vi "CRYGet Harmonics Curve array.vi"(4 "Impedance and Mic Current In":bool[](array[boolean]), 5 "Additive Info":T4, 6 "Option Array In":bool[](array[boolean]), 7 "Unit Info":T5, 8 "Diff array":dbl[](array[numeric]), 9 "IM array":dbl[](array[numeric]), 10 "Harmonics array":dbl[](array[numeric]), 11 "Type":u16) -> (0 "Display Array":T3(array[cluster]), 1 "Unit Info Out":T2[](array[typedef]), 2 "Harmonics Orders Out":dbl[](array[numeric]), 3 "Curve Info Array Out":T1)   [LabVIEW 2013]
uses:
  Typedef Control/CRYUnit Info Cluster.ctl
  Typedef Control/CRYUnit Info Out Cluster.ctl
  Typedef Control/CRYAnalysis CurveName Cluster.ctl
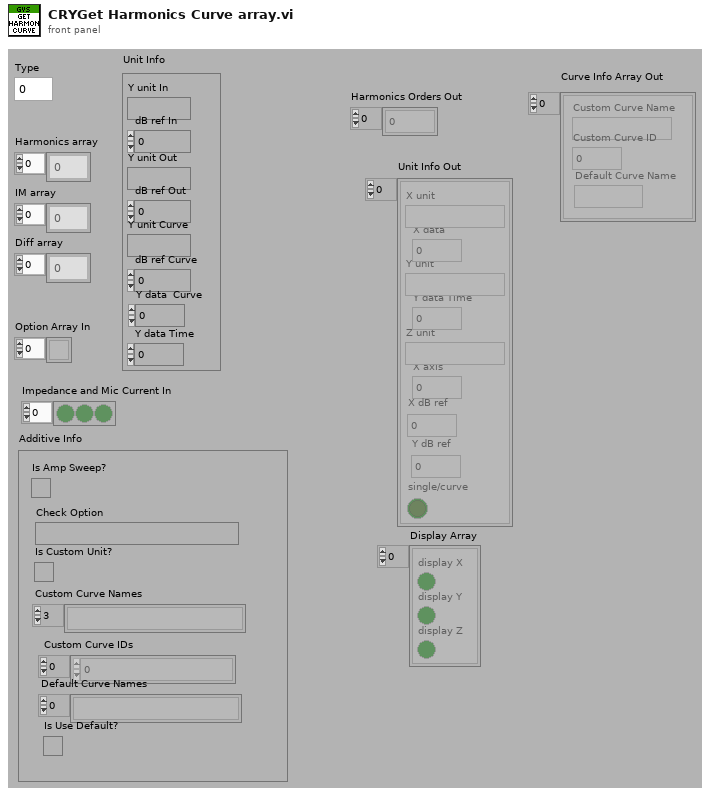
[diagram p1: front panel]
types:
  T1 = typedef "CRYAnalysis CurveName Cluster.ctl" = cluster{"Custom Curve Name":string, "Custom Curve ID":i32, "Default Curve Name":string}[]
  T2 = typedef "CRYUnit Info Out Cluster.ctl" = cluster{"X unit":string, "X data":u16, "Y unit":string, "Y data Time":u16, "Z unit":string, "X axis":u16, "X dB ref":dbl, "Y dB ref":dbl, "single/curve":bool}
  T3 = cluster{"display X":bool, "display Y":bool, "display Z":bool}[]
  T4 = cluster{"Is Amp Sweep?":bool, "Check Option":string, "Is Custom Unit?":bool, "Custom Curve Names":string[], "Custom Curve IDs":i32[], "Default Curve Names":string[], "Is Use Default?":bool}
  T5 = typedef "CRYUnit Info Cluster.ctl" = cluster{"Y unit In":string, "dB ref In":dbl, "Y unit Out":string, "dB ref Out":dbl, "Y unit Curve":string, "dB ref Curve":dbl, "Y data  Curve":u16, "Y data Time":u16}
  T6 = enum32{"English", "Chinese", "Korean", "Japanese", "Russian", "Chinese traditional"}
  T7 = cluster{"Y unit Out":string, "dB":u16, "Y unit Curve":string, "Y data  Curve":u16, "Y unit Curve":string, "Lin":u16, "dB ref Out":dbl, "dB ref Curve":dbl, "display X":bool}
  T8 = cluster{"display X":bool, "display Y":bool, "display Z":bool}
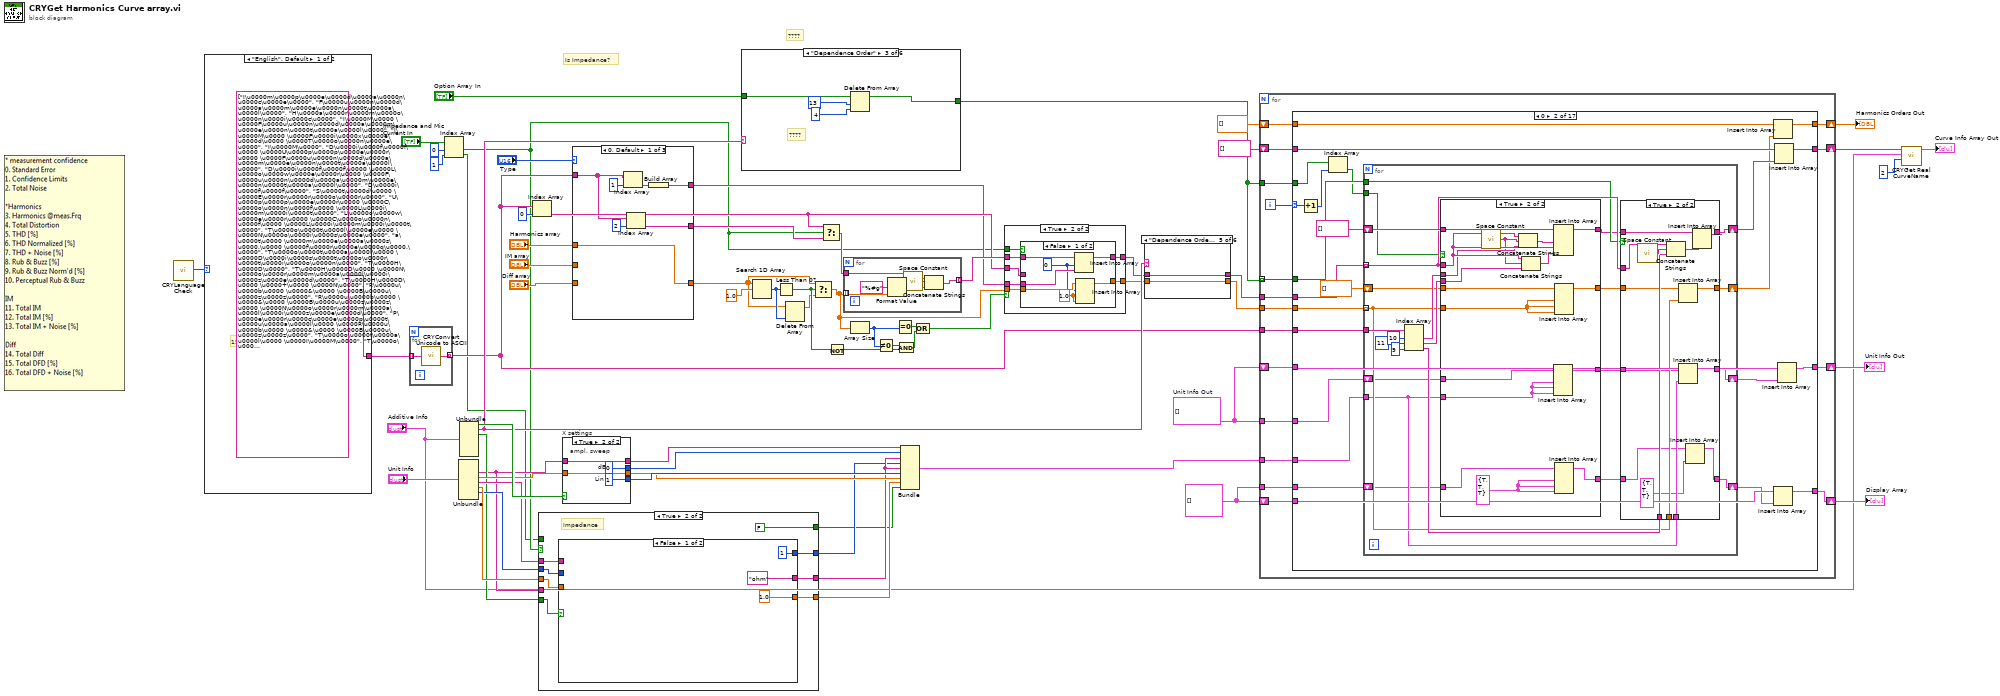
[diagram p0: block diagram]
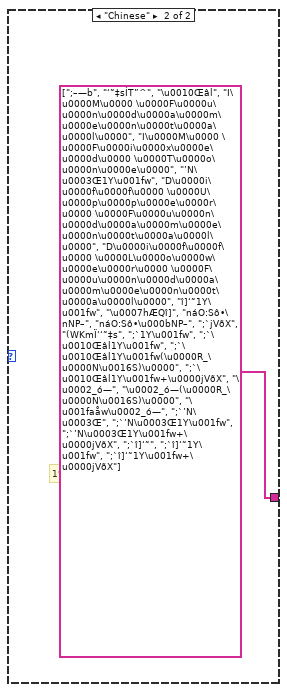
[diagram p2: hidden frame]
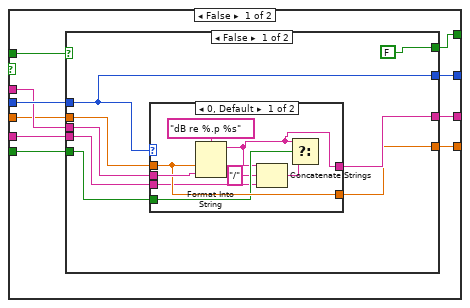
[diagram p3: hidden frame]
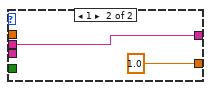
[diagram p4: hidden frame]
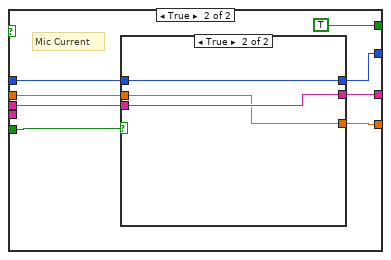
[diagram p5: hidden frame]
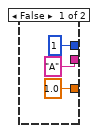
[diagram p6: hidden frame]
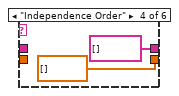
[diagram p11: hidden frame]
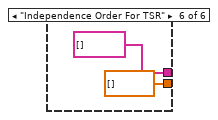
[diagram p12: hidden frame]
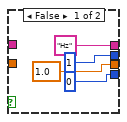
[diagram p13: hidden frame]
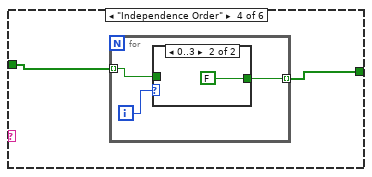
[diagram p16: hidden frame]
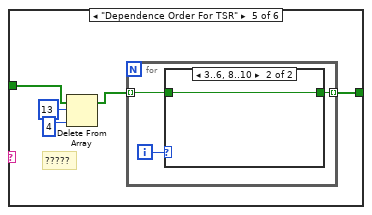
[diagram p18: hidden frame]
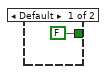
[diagram p19: hidden frame]
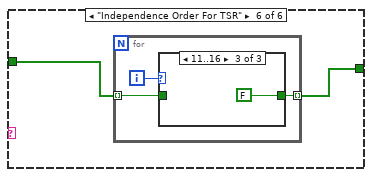
[diagram p20: hidden frame]
diagram:
  w28 = T3 [] ("Display Array")
  w31 = T2[] []  # Unit Info Out
  # "????"
  # "Is Impedance?"
  n1 = call "CRYLanguage Check.vi"() -> ("Language"=w8:T6)  [unwired: 10 in, 1 out]
  n2 = case shown="\"English\", Default" w8 {
    tunnel: [string[] ["I\u0000m\u0000p\u0000e\u0000d\u0000a\u0000n\u0000c\u0000e\u0000", "F\u0000u\u0000n\u0000d\u0000a\u0000m\u0000e\u0000n\u0000t\u0000a\u0000l\u0000", "H\u0000a\u0000r\u0000m\u0000o\u0000n\u0000i\u0000c\u0000", "I\u0000M\u0000 \u0000F\u0000u\u0000n\u0000d\u0000a\u0000m\u0000e\u0000n\u0000t\u0000a\u0000l\u0000", "I\u0000M\u0000 \u0000F\u0000i\u0000x\u0000e\u0000d\u0000 \u0000T\u0000o\u0000n\u0000e\u0000", "I\u0000M\u0000", "D\u0000i\u0000f\u0000f\u0000 \u0000U\u0000p\u0000p\u0000e\u0000r\u0000 \u0000F\u0000u\u0000n\u0000d\u0000a\u0000m\u0000e\u0000n\u0000t\u0000a\u0000l\u0000", "D\u0000i\u0000f\u0000f\u0000 \u0000L\u0000o\u0000w\u0000e\u0000r\u0000 \u0000F\u0000u\u0000n\u0000d\u0000a\u0000m\u0000e\u0000n\u0000t\u0000a\u0000l\u0000", "D\u0000i\u0000f\u0000f\u0000", "S\u0000t\u0000d\u0000 \u0000E\u0000r\u0000r\u0000o\u0000r\u0000", "U\u0000p\u0000p\u0000e\u0000r\u0000 \u0000C\u0000o\u0000n\u0000f\u0000 \u0000L\u0000i\u0000m\u0000i\u0000t\u0000", "L\u0000o\u0000w\u0000e\u0000r\u0000 \u0000C\u0000o\u0000n\u0000f\u0000 \u0000L\u0000i\u0000m\u0000i\u0000t\u0000", "T\u0000o\u0000t\u0000l\u0000e\u0000 \u0000N\u0000o\u0000i\u0000s\u0000e\u0000", "a\u0000t\u0000 \u0000m\u0000e\u0000a\u0000s\u0000.\u0000 \u0000f\u0000r\u0000e\u0000q\u0000.\u0000", "T\u0000o\u0000t\u0000a\u0000l\u0000 \u0000D\u0000i\u0000s\u0000t\u0000o\u0000r\u0000t\u0000i\u0000o\u0000n\u0000", "T\u0000H\u0000D\u0000", "T\u0000H\u0000D\u0000 \u0000N\u0000o\u0000r\u0000m\u0000a\u0000l\u0000i\u0000z\u0000e\u0000d\u0000", "T\u0000H\u0000D\u0000 \u0000+\u0000 \u0000N\u0000", "R\u0000u\u0000b\u0000 \u0000&\u0000 \u0000B\u0000u\u0000z\u0000z\u0000", "R\u0000u\u0000b\u0000 \u0000&\u0000 \u0000B\u0000u\u0000z\u0000z\u0000 \u0000N\u0000o\u0000r\u0000m\u0000a\u0000l\u0000i\u0000z\u0000e\u0000d\u0000", "P\u0000e\u0000r\u0000c\u0000e\u0000p\u0000t\u0000u\u0000a\u0000l\u0000 \u0000R\u0000u\u0000b\u0000 \u0000&\u0000 \u0000B\u0000u\u0000z\u0000z\u0000", "T\u0000o\u0000t\u0000a\u0000l\u0000 \u0000I\u0000M\u0000", "T\u0000o\u0000t\u0000a\u0000l\u0000 \u0000I\u0000M\u0000D\u0000", "T\u0000o\u0000t\u0000a\u0000l\u0000 \u0000I\u0000M\u0000D\u0000 \u0000+\u0000 \u0000N\u0000", "T\u0000o\u0000t\u0000a\u0000l\u0000 \u0000D\u0000i\u0000f\u0000f\u0000", "T\u0000o\u0000t\u0000a\u0000l\u0000 \u0000D\u0000F\u0000D\u0000", "T\u0000o\u0000t\u0000a\u0000l\u0000 \u0000D\u0000F\u0000D\u0000 \u0000+\u0000 \u0000N\u0000"] ("Array") string[] [";–—b", "‘˜‡sÍT”^", "\u0010Œâl", "I\u0000M\u0000 \u0000F\u0000u\u0000n\u0000d\u0000a\u0000m\u0000e\u0000n\u0000t\u0000a\u0000l\u0000", "I\u0000M\u0000 \u0000F\u0000i\u0000x\u0000e\u0000d\u0000 \u0000T\u0000o\u0000n\u0000e\u0000", "’N\u0003Œ1Y\u001fw", "D\u0000i\u0000f\u0000f\u0000 \u0000U\u0000p\u0000p\u0000e\u0000r\u0000 \u0000F\u0000u\u0000n\u0000d\u0000a\u0000m\u0000e\u0000n\u0000t\u0000a\u0000l\u0000", "D\u0000i\u0000f\u0000f\u0000 \u0000L\u0000o\u0000w\u0000e\u0000r\u0000 \u0000F\u0000u\u0000n\u0000d\u0000a\u0000m\u0000e\u0000n\u0000t\u0000a\u0000l\u0000", "î]‘˜1Y\u001fw", "\u0007hÆQî]", "náO:Sô•\nNP–", "náO:Sô•\u000bNP–", ";`jVðX", "(WKmÏ‘‘˜‡s", ";`1Y\u001fw", ";`\u0010Œâl1Y\u001fw", ";`\u0010Œâl1Y\u001fw(\u0000R_\u0000N\u0016S)\u0000", ";`\u0010Œâl1Y\u001fw+\u0000jVðX", "\u0002_ó—", "\u0002_ó—(\u0000R_\u0000N\u0016S)\u0000", "\u001faåw\u0002_ó—", ";`’N\u0003Œ", ";`’N\u0003Œ1Y\u001fw", ";`’N\u0003Œ1Y\u001fw+\u0000jVðX", ";`î]‘˜", ";`î]‘˜1Y\u001fw", ";`î]‘˜1Y\u001fw+\u0000jVðX"] ("Array")] -> w10
    frame "English", Default {
      # "19"
    }
    frame "Chinese" {
      # "19"
    }
  }
  n3 = for {
    tunnel: w10 -> [w69] mode=indexing
    tunnel: [w68] -> w9 mode=indexing
    n4 = call "CRYConvert Unicode to ASCII.vi"("Unicode"=w69) -> ("ASCII"=w68:string)  [unwired: 4 in]
  }
  n5 = Index Array(array="Impedance and Mic Current In", index #1=0 ("index"), index #2=1 ("index")) -> (element #1=w4:bool, element #2=w2:bool)
  n6 = Unbundle("Unit Info") -> ("Y unit Out"=w15:string, "dB ref Out"=w37:dbl, "Y unit Curve"=w20:string, "dB ref Curve"=w19:dbl, "Y data  Curve"=w17:u16)  [unwired: 3 out]
  n7 = Unbundle("Additive Info") -> ("Is Amp Sweep?"=w38:bool, "Check Option"=w26:string, "Is Custom Unit?"=w16:bool)  [unwired: 4 out]
  n8 = Index Array(array=w9, index=0) -> (element=w50:string)
  n9 = case shown="True" w4 {
    tunnel: w20 -> [w77 w114]
    tunnel: [w78 w119] -> w21
    tunnel: w17 -> [w79 w116]
    tunnel: w19 -> [w76 w113]
    tunnel: [w75 w118] -> w18
    tunnel: w16 -> [w74 w117]
    tunnel: w15 -> [w73 _]
    tunnel: [w71 w115] -> w3
    tunnel: w2 -> [w72 _]
    tunnel: [w70 FALSE ("display X")] -> w1
    frame False {
      n10 = case shown="False" w72 {
        tunnel: w79 -> [w81 w103]
        tunnel: [w87 w102] -> w78
        tunnel: w77 -> [w86 w101]
        tunnel: w76 -> [w85 w99]
        tunnel: [w84 w100] -> w75
        tunnel: w74 -> [w83 w105]
        tunnel: w73 -> [w82 _]
        tunnel: [w81 w104] -> w71
        tunnel: [FALSE ("display X") TRUE ("display X")] -> w70
        frame False {
          n11 = case shown="0, Default" w81 {
            tunnel: [w88 w96] -> w87
            tunnel: w85 -> [w93 _]
            tunnel: w86 -> [w94 w96]
            tunnel: [w93 1.0 ("dB ref Curve")] -> w84
            tunnel: w83 -> [w92 _]
            tunnel: w82 -> [w89 _]
            frame 0, Default {
              n12 = Format Into String(format string="dB re %.p %s", w93, w94) -> (resulting string=w88:string)  [unwired: 2 in, 1 out]
              n13 = Concatenate Strings(w88, "/" ("string"), w89) -> (w91:string)
              n14 = Select(t=w88, s=w92, f=w91) -> ()  [unwired: 1 out]
            }
            frame 1 {
            }
          }
        }
        frame True {
          # "Mic Current"
          n15 = case shown="True" w105 {
            tunnel: [u16 1 ("Y data  Curve") w111] -> w104
            tunnel: w103 -> [_ w111]
            tunnel: ["A" ("Y unit Curve") w110] -> w102
            tunnel: w101 -> [_ w110]
            tunnel: [1.0 ("dB ref Curve") w109] -> w100
            tunnel: w99 -> [_ w109]
            frame False {
            }
            frame True {
            }
          }
        }
      }
    }
    frame True {
      # "Impedance"
      n16 = case shown="False" w117 {
        tunnel: ["ohm" ("unit") w124] -> w119
        tunnel: [1.0 ("dB ref Curve") w123] -> w118
        tunnel: [u16 1 ("Y data  Curve") w125] -> w115
        tunnel: w116 -> [_ w125]
        tunnel: w114 -> [_ w124]
        tunnel: w113 -> [_ w123]
        frame False {
        }
        frame True {
        }
      }
    }
  }
  n17 = case "X settings" shown="True" w38 {
    tunnel: ["Hz" ("X unit") w131] -> w36
    tunnel: [u16 1 ("Y data") w132] -> w35
    tunnel: [1.0 ("X dB ref") w130] -> w33
    tunnel: [u16 0 ("X axis") w133] -> w34
    tunnel: w15 -> [_ w131]
    tunnel: w37 -> [_ w130]
    frame False {
    }
    frame True {
      w132 = u16 0  # dB
      w133 = u16 1  # Lin
      # "ampl. sweep"
    }
  }
  n18 = case shown="0, Default" "Type" {
    tunnel: [w134 w141 w148] -> w52
    tunnel: w9 -> [w135 w142 w149]
    tunnel: [w138 w145 w152] -> w49
    tunnel: [w136 w144 w151] -> w48
    tunnel: "Harmonics array" -> [w134 _ _]
    tunnel: "Diff array" -> [_ _ w148]
    tunnel: "IM array" -> [_ w141 _]
    frame 0, Default {
      n19 = Index Array(array=w135, index=1) -> (element=w139:string)
      n20 = Index Array(array=w135, index=2) -> (element=w136:string)
      n21 = Build Array(w139) -> (w138:string[])
    }
    frame 1 {
      n22 = Array Subset(array=w142, index=3, length=2) -> (w145:string[])
      n23 = Index Array(array=w142, index=5) -> (element=w144:string)
    }
    frame 2 {
      n24 = Index Array(array=w149, index=8) -> (element=w151:string)
      n25 = Array Subset(array=w149, index=6, length=2) -> (w152:string[])
    }
  }
  n26 = case shown="\"Dependence Order\"" w26 {
    tunnel: "Option Array In" -> [w155 w156 w158 w162 w169 w179]
    tunnel: [w155 w156 w157 w161 w172 w178] -> w39
    frame Default {
    }
    frame "All" {
    }
    frame "Dependence Order" {
      # "????"
      n27 = Delete From Array(array=w158, length=13, index=4) -> (array with subset deleted=w157:bool[])  [unwired: 1 out]
    }
    frame "Independence Order" {
      n28 = for {
        tunnel: w162 -> [w164] mode=indexing
        tunnel: [w163] -> w161 mode=indexing
        i -> [w165]
        n29 = case shown="0..3" w165 {
          tunnel: w164 -> [w166 _]
          tunnel: [w166 FALSE ("Total DFD+Noise(%)")] -> w163
          frame Default {
          }
          frame 0..3 {
          }
        }
      }
    }
    frame "Dependence Order For TSR" {
      # "?????"
      n30 = Delete From Array(array=w169, length=13, index=4) -> (array with subset deleted=w168:bool[])  [unwired: 1 out]
      n31 = for {
        tunnel: w168 -> [w174] mode=indexing
        tunnel: [w173] -> w172 mode=indexing
        i -> [w175]
        n32 = case shown="3..6, 8..10" w175 {
          tunnel: w174 -> [_ w177]
          tunnel: [FALSE ("Is Har meas.freq? 2") w177] -> w173
          frame Default {
          }
          frame 3..6, 8..10 {
          }
        }
      }
    }
    frame "Independence Order For TSR" {
      n33 = for {
        tunnel: w179 -> [w181] mode=indexing
        tunnel: [w180] -> w178 mode=indexing
        i -> [w182]
        n34 = case shown="11..16" w182 {
          tunnel: w181 -> [w183 _ _]
          tunnel: [w183 FALSE ("Is Har meas.freq? 2") FALSE ("Is Har meas.freq? 2")] -> w180
          frame Default {
          }
          frame 0..3, 7 {
          }
          frame 11..16 {
          }
        }
      }
    }
  }
  n35 = Search 1D Array(1D array=w52, element=1.0) -> (index of element=w58:i32)  [unwired: 1 out]
  n36 = Less Than 0?(x=w58) -> (x < 0?=w63:bool)
  n37 = Delete From Array(array=w52, index=w58) -> (array with subset deleted=w59:dbl[])  [unwired: 1 in, 1 out]
  n38 = Select(t=w52, s=w63, f=w59) -> (s? t:f=w43:dbl[])
  n39 = Select(t=w50, s=w4, f=w48) -> (s? t:f=w56:string)
  n40 = Not(x=w63) -> (.not. x?=w64:bool)
  n41 = for {
    tunnel: w43 -> [w190] mode=indexing
    tunnel: [w188] -> w54 mode=indexing
    tunnel: w56 -> [w187]
    n42 = Format Value(format string="%#g", value (0)=w190) -> (output string=w189:string)  [unwired: 1 out]
    n43 = call <vilib>:"Space Constant.vi"() -> ("String"=w186:string)
    n44 = Concatenate Strings(w187, w186, w189) -> (w188:string)
  }
  n45 = Array Size(array=w43) -> (size(s)=w61:i32)
  n46 = Not Equal To 0?(x=w61) -> (x != 0?=w62:bool)
  n47 = Equal To 0?(x=w61) -> (x = 0?=w60:bool)
  n48 = And(x=w62, y=w64) -> (x .and. y?=w65:bool)
  n49 = Bundle("Y unit Out"=w36, "dB"=w35, "Y unit Curve"=w21, "Y data  Curve"=w3, "Y unit Curve"=w21, "Lin"=w34, "dB ref Out"=w33, "dB ref Curve"=w18, "display X"=w1) -> (w29:T7)  [unwired: 1 in]
  n50 = Or(x=w60, y=w65) -> (x .or. y?=w55:bool)
  n51 = case shown="True" w55 {
    tunnel: w54 -> [w193 w200]
    tunnel: [w193 w199] -> w25
    tunnel: w4 -> [_ w198]
    tunnel: w50 -> [_ w197]
    tunnel: w49 -> [_ w196]
    tunnel: w43 -> [w192 w195]
    tunnel: [w192 w194] -> w24
    frame False {
    }
    frame True {
      n52 = case shown="False" w198 {
        tunnel: w200 -> [w207 w214]
        tunnel: [w206 w213] -> w199
        tunnel: w197 -> [_ w212]
        tunnel: w196 -> [w205 _]
        tunnel: w195 -> [w204 w211]
        tunnel: [w201 w210] -> w194
        frame False {
          w202 = 1.0 ("new element/subarray")
          w203 = 0 ("index")
          n53 = Insert Into Array(array=w207, index=w203, new element=w205) -> (w206:string[])
          n54 = Insert Into Array(array=w204, index=w203, new element #1=w202, new element #2=w202) -> (w201:dbl[])
        }
        frame True {
          w209 = 0 ("index")
          n55 = Insert Into Array(array=w211, index=w209, new element=1.0 ("new element/subarray")) -> (w210:dbl[])
          n56 = Insert Into Array(array=w214, index=w209, new element=w212) -> (w213:string[])
        }
      }
    }
  }
  n57 = case shown="\"Dependence Order For TSR\"" w26 {
    tunnel: w25 -> [w216 w218 w220 _ w224 _]
    tunnel: w24 -> [w215 w217 w219 _ w223 _]
    tunnel: [w216 w218 w220 string[] [] w224 string[] []] -> w23
    tunnel: [w215 w217 w219 dbl[] [] ("Diff array") w223 dbl[] [] ("Diff array")] -> w22
    frame Default {
    }
    frame "All" {
    }
    frame "Dependence Order" {
    }
    frame "Independence Order" {
    }
    frame "Dependence Order For TSR" {
    }
    frame "Independence Order For TSR" {
    }
  }
  n58 = for {
    tunnel: w39 -> [w241] mode=indexing
    shift-right: [w242] -> w14
    shift-left: string[] [] ("Array") -> [w243]
    tunnel: w23 -> [w239]
    tunnel: w39 -> [w238]
    tunnel: w9 -> [w237]
    tunnel: w22 -> [w236]
    shift-right: [w234] -> w41
    shift-left: dbl[] [] ("Diff array") -> [w235]
    tunnel: w29 -> [w232]
    shift-right: [w230] -> w30
    shift-left: w31 -> [w231]
    tunnel: w31 -> [w233]
    shift-right: [w228] -> w27
    shift-left: w28 -> [w229]
    tunnel: w28 -> [w227]
    i -> [w240]
    n59 = case shown="0" w240 {
      selector: w240 -> [_ w269 _ _ w442 w476 w510 w544 w579 w614 w649 w684 w718 w753 w788 w822 w857]
      tunnel: w243 -> [w247 w263 w357 w386 w446 w480 w514 w548 w583 w618 w653 w688 w722 w757 w792 w826 w861]
      tunnel: [w247 w264 w356 w385 w443 w477 w511 w545 w580 w615 w650 w685 w719 w754 w789 w823 w858] -> w242
      tunnel: w241 -> [_ w271 w355 w391 w445 w479 w513 w547 w582 w617 w652 w687 w721 w756 w791 w825 w860]
      tunnel: w239 -> [_ w272 _ w390 _ _ _ _ _ _ _ _ _ _ _ _ _]
      tunnel: w238 -> [_ w270 _ _ _ _ _ _ _ _ _ _ _ _ _ _ _]
      tunnel: w237 -> [_ w266 w354 w388 w444 w478 w512 w546 w581 w616 w651 w686 w720 w755 w790 w824 w859]
      tunnel: w236 -> [_ w261 _ w383 _ _ _ _ _ _ _ _ _ _ _ _ _]
      tunnel: w235 -> [w246 w260 w351 w380 w439 w473 w507 w541 w576 w611 w646 w681 w715 w750 w785 w819 w854]
      tunnel: [w246 w259 w350 w379 w439 w473 w507 w541 w576 w611 w646 w681 w715 w750 w785 w819 w854] -> w234
      tunnel: w233 -> [_ w256 _ _ _ _ _ _ _ _ _ _ _ _ _ _ _]
      tunnel: w232 -> [_ w255 w348 w377 w437 w471 w505 w539 w574 w609 w644 w679 w713 w748 w783 w817 w852]
      tunnel: w231 -> [w245 w254 w349 w378 w438 w472 w506 w540 w575 w610 w645 w680 w714 w749 w784 w818 w853]
      tunnel: [w245 w252 w347 w376 w436 w470 w504 w538 w573 w608 w643 w678 w712 w747 w782 w816 w851] -> w230
      tunnel: w229 -> [w244 w250 w346 w375 w435 w469 w503 w537 w572 w607 w642 w677 w711 w746 w781 w815 w850]
      tunnel: [w244 w251 w345 w374 w434 w468 w502 w536 w571 w606 w641 w676 w710 w745 w780 w814 w849] -> w228
      tunnel: w227 -> [_ w249 _ _ _ _ _ _ _ _ _ _ _ _ _ _ _]
      frame Default {
      }
      frame 0 {
        n60 = Increment(x=w269) -> (x+1=w268:i32)
        n61 = Index Array(array=w270, index=w268) -> (element=w267:bool)
        n62 = for {
          tunnel: w272 -> [w294] mode=indexing
          tunnel: w267 -> [w293]
          shift-right: [w295] -> w262
          shift-left: string[] [] ("Array") -> [w296]
          tunnel: w271 -> [w292]
          tunnel: w266 -> [w287]
          tunnel: w261 -> [w281] mode=indexing
          shift-right: [w280] -> w257
          shift-left: dbl[] [] ("Diff array") -> [w283]
          shift-right: [w276] -> w253
          shift-left: w256 -> [w279]
          tunnel: w255 -> [w277]
          shift-right: [w273] -> w248
          shift-left: w249 -> [w275]
          n63 = Index Array(array=w287, index #1=10 ("index"), index #2=11 ("index"), index #3=9 ("index")) -> (element #1=w284:string, element #2=w285:string, element #3=w286:string)
          n64 = case shown="True" w293 {
            tunnel: w294 -> [w325 w341]
            tunnel: w296 -> [w327 w343]
            tunnel: [w326 w342] -> w291
            tunnel: w284 -> [_ w339]
            tunnel: w285 -> [_ w338]
            tunnel: w283 -> [w324 w336]
            tunnel: w281 -> [w322 w335]
            tunnel: [w323 w334] -> w282
            tunnel: w279 -> [w321 w333]
            tunnel: w277 -> [w319 w332]
            tunnel: [w320 w331] -> w278
            tunnel: w275 -> [w318 w330]
            tunnel: [w317 w329] -> w274
            frame False {
              n65 = Insert Into Array(array=w327, new element=w325) -> (w326:string[])  [unwired: 1 in]
              n66 = Insert Into Array(array=w324, new element=w322) -> (w323:dbl[])  [unwired: 1 in]
              n67 = Insert Into Array(array=w318, new element=T8 {"display X"=TRUE, "display Y"=TRUE, "display Z"=TRUE}) -> (w317:T3)  [unwired: 1 in]
              n68 = Insert Into Array(array=w321, new element=w319) -> (w320:T2[])  [unwired: 1 in]
            }
            frame True {
              w328 = T8 {"display X"=TRUE, "display Y"=TRUE, "display Z"=TRUE}
              n69 = call <vilib>:"Space Constant.vi"() -> ("String"=w337:string)
              n70 = Concatenate Strings(w341, w337, w339) -> (w344:string)
              n71 = Concatenate Strings(w341, w337, w338) -> (w340:string)
              n72 = Insert Into Array(array=w333, new element #1=w332, new element #2=w332, new element #3=w332) -> (w331:T2[])  [unwired: 1 in]
              n73 = Insert Into Array(array=w343, new element #1=w344, new element #2=w341, new element #3=w340) -> (w342:string[])  [unwired: 1 in]
              n74 = Insert Into Array(array=w336, new element #1=w335, new element #2=w335, new element #3=w335) -> (w334:dbl[])  [unwired: 1 in]
              n75 = Insert Into Array(array=w330, new element #1=w328, new element #2=w328, new element #3=w328) -> (w329:T3)  [unwired: 1 in]
            }
          }
          n76 = case shown="True" w292 {
            tunnel: w291 -> [w300 w315]
            tunnel: [w300 w312] -> w295
            tunnel: w294 -> [_ w314]
            tunnel: w286 -> [_ w310]
            tunnel: w282 -> [w299 w309]
            tunnel: [w299 w308] -> w280
            tunnel: w281 -> [_ w307]
            tunnel: w278 -> [w298 w306]
            tunnel: w277 -> [_ w305]
            tunnel: [w298 w304] -> w276
            tunnel: w274 -> [w297 w303]
            tunnel: [w297 w302] -> w273
            frame False {
            }
            frame True {
              n77 = call <vilib>:"Space Constant.vi"() -> ("String"=w311:string)
              n78 = Concatenate Strings(w314, w311, w310) -> (w313:string)
              n79 = Insert Into Array(array=w309, new element=w307) -> (w308:dbl[])  [unwired: 1 in]
              n80 = Insert Into Array(array=w306, new element=w305) -> (w304:T2[])  [unwired: 1 in]
              n81 = Insert Into Array(array=w303, new element=T8 {"display X"=TRUE, "display Y"=TRUE, "display Z"=TRUE}) -> (w302:T3)  [unwired: 1 in]
              n82 = Insert Into Array(array=w315, new element=w313) -> (w312:string[])  [unwired: 1 in]
            }
          }
        }
        n83 = Insert Into Array(array=w260, new element=w257) -> (w259:dbl[])  [unwired: 1 in]
        n84 = Insert Into Array(array=w250, new element=w248) -> (w251:T3)  [unwired: 1 in]
        n85 = Insert Into Array(array=w263, new element=w262) -> (w264:string[])  [unwired: 1 in]
        n86 = Insert Into Array(array=w254, new element=w253) -> (w252:T2[])  [unwired: 1 in]
      }
      frame 2 {
        n87 = Index Array(array=w354, index=12) -> (element=w352:string)
        n88 = case shown="True" w355 {
          tunnel: w357 -> [w361 w373]
          tunnel: w352 -> [_ w372]
          tunnel: [w361 w371] -> w356
          tunnel: w351 -> [w360 w370]
          tunnel: [w360 w369] -> w350
          tunnel: w349 -> [w359 w367]
          tunnel: w348 -> [_ w366]
          tunnel: [w359 w365] -> w347
          tunnel: w346 -> [w358 w364]
          tunnel: [w358 w363] -> w345
          frame False {
          }
          frame True {
            n89 = Insert Into Array(array=w373, new element=w372) -> (w371:string[])  [unwired: 1 in]
            n90 = Insert Into Array(array=w370, new element=1.0 ("new element/subarray")) -> (w369:dbl[])  [unwired: 1 in]
            n91 = Insert Into Array(array=w367, new element=w366) -> (w365:T2[])  [unwired: 1 in]
            n92 = Insert Into Array(array=w364, new element=T8 {"display X"=TRUE, "display Y"=TRUE, "display Z"=TRUE}) -> (w363:T3)  [unwired: 1 in]
          }
        }
      }
      frame 3 {
        n93 = Index Array(array=w388, index=13) -> (element=w387:string)
        n94 = for {
          tunnel: w383 -> [w400] mode=indexing
          tunnel: [w397] -> w382
          tunnel: [w396] -> w384
          i -> [w397]
          stop <- w396 stop-if-true
          n95 = Greater?(x=w400, y=0.9999) -> (0:w399:bool)
          n96 = Less?(x=w400, y=1.00001) -> (x < y?=w398:bool)
          n97 = And(x=w399, y=w398) -> (x .and. y?=w396:bool)
        }
        n98 = case shown="True" w384 {
          tunnel: w383 -> [w392 w395]
          tunnel: w382 -> [_ w394]
          tunnel: [w392 w393] -> w381
          frame False {
          }
          frame True {
            n99 = Delete From Array(array=w395, index=w394) -> (array with subset deleted=w393:dbl[])  [unwired: 1 in, 1 out]
          }
        }
        n100 = case shown="True" w391 {
          tunnel: w390 -> [_ w422]
          tunnel: w387 -> [_ w420]
          tunnel: w386 -> [w406 w419]
          tunnel: [w406 w418] -> w385
          tunnel: w381 -> [_ w416]
          tunnel: [w405 w415] -> w379
          tunnel: w380 -> [w405 w417]
          tunnel: w378 -> [w404 w413]
          tunnel: [w404 w412] -> w376
          tunnel: w377 -> [_ w414]
          tunnel: w375 -> [w403 w409]
          tunnel: [w403 w407] -> w374
          frame False {
          }
          frame True {
            n101 = Array Size(array=w422) -> (size(s)=w424:i32)
            n102 = Decrement(x=w424) -> (x-1=w423:i32)
            n103 = for {
              N: w423 -> [_]
              tunnel: w422 -> [w433]
              tunnel: [w429] -> w421 mode=indexing
              tunnel: w420 -> [w427]
              tunnel: w414 -> [w426]
              tunnel: [w426] -> w411 mode=indexing
              tunnel: T8 {"display X"=TRUE, "display Y"=TRUE, "display Z"=TRUE} -> [w425]
              tunnel: [w425] -> w408 mode=indexing
              i -> [w432]
              n104 = Increment(x=w432) -> (x+1=w431:i32)
              n105 = Index Array(array=w433, index=w431) -> (element=w430:string)
              n106 = call <vilib>:"Space Constant.vi"() -> ("String"=w428:string)
              n107 = Concatenate Strings(w430, w428, w427) -> (w429:string)
            }
            n108 = Insert Into Array(array=w417, new element=w416) -> (w415:dbl[])  [unwired: 1 in]
            n109 = Insert Into Array(array=w413, new element=w411) -> (w412:T2[])  [unwired: 1 in]
            n110 = Insert Into Array(array=w409, new element=w408) -> (w407:T3)  [unwired: 1 in]
            n111 = Insert Into Array(array=w419, new element=w421) -> (w418:string[])  [unwired: 1 in]
          }
        }
      }
      frame 4 {
        n112 = Add(x=w442, y=10) -> (x+y=w440:i32)
        n113 = Index Array(array=w444, index=w440) -> (element=w447:string)
        n114 = case shown="True" w445 {
          tunnel: w446 -> [w450 w467]
          tunnel: w447 -> [_ w466]
          tunnel: [w450 w465] -> w443
          tunnel: w438 -> [w449 w464]
          tunnel: w437 -> [_ w451]
          tunnel: [w449 w463] -> w436
          tunnel: w435 -> [w448 w454]
          tunnel: [w448 w453] -> w434
          frame False {
          }
          frame True {
            n115 = Unbundle(w451) -> ("dB"=w458:u16, "Y unit Curve"=w462:string, "Lin"=w457:u16, "dB ref Out"=w456:dbl, "dB ref Curve"=w455:dbl)  [unwired: 4 out]
            n116 = Insert Into Array(array=w467, new element=w466) -> (w465:string[])  [unwired: 1 in]
            n117 = Bundle(cluster=w451, "Y unit Out"="Hz" ("X unit"), "dB"=w458, "Y unit Curve"=w462, "Y data  Curve"=u16 1 ("Y data"), "Y unit Curve"="deg." ("Z unit"), "Lin"=w457, "dB ref Out"=w456, "dB ref Curve"=w455) -> ()  [unwired: 1 in, 1 out]
            n118 = Insert Into Array(array=w454, new element=T8 {"display X"=TRUE, "display Y"=TRUE, "display Z"=TRUE}) -> (w453:T3)  [unwired: 1 in]
            n119 = Insert Into Array(array=w464, new element=w451) -> (w463:T2[])  [unwired: 1 in]
          }
        }
      }
      frame 5 {
        n120 = Add(x=w476, y=10) -> (x+y=w474:i32)
        n121 = Index Array(array=w478, index=w474) -> (element=w481:string)
        n122 = case shown="True" w479 {
          tunnel: w480 -> [w484 w501]
          tunnel: w481 -> [_ w500]
          tunnel: [w484 w499] -> w477
          tunnel: w472 -> [w483 w498]
          tunnel: w471 -> [_ w495]
          tunnel: [w483 w497] -> w470
          tunnel: w469 -> [w482 w488]
          tunnel: [w482 w487] -> w468
          frame False {
          }
          frame True {
            n123 = Unbundle(w495) -> ("dB"=w492:u16, "Lin"=w491:u16, "dB ref Out"=w490:dbl, "dB ref Curve"=w489:dbl)  [unwired: 5 out]
            n124 = Insert Into Array(array=w501, new element=w500) -> (w499:string[])  [unwired: 1 in]
            n125 = Bundle(cluster=w495, "Y unit Out"="Hz" ("X unit"), "dB"=w492, "Y unit Curve"="%" ("Y unit"), "Y data  Curve"=u16 1 ("Y data"), "Lin"=w491, "dB ref Out"=w490, "dB ref Curve"=w489) -> (w496:T7)  [unwired: 2 in]
            n126 = Insert Into Array(array=w488, new element=T8 {"display X"=TRUE, "display Y"=TRUE, "display Z"=FALSE}) -> (w487:T3)  [unwired: 1 in]
            n127 = Insert Into Array(array=w498, new element=w496) -> (w497:T2[])  [unwired: 1 in]
          }
        }
      }
      frame 6 {
        n128 = Add(x=w510, y=10) -> (x+y=w508:i32)
        n129 = Index Array(array=w512, index=w508) -> (element=w515:string)
        n130 = case shown="True" w513 {
          tunnel: w514 -> [w518 w535]
          tunnel: w515 -> [_ w534]
          tunnel: [w518 w533] -> w511
          tunnel: w506 -> [w517 w532]
          tunnel: w505 -> [_ w529]
          tunnel: [w517 w531] -> w504
          tunnel: w503 -> [w516 w522]
          tunnel: [w516 w521] -> w502
          frame False {
          }
          frame True {
            n131 = Unbundle(w529) -> ("dB"=w526:u16, "Lin"=w525:u16, "dB ref Out"=w524:dbl, "dB ref Curve"=w523:dbl)  [unwired: 5 out]
            n132 = Insert Into Array(array=w535, new element=w534) -> (w533:string[])  [unwired: 1 in]
            n133 = Bundle(cluster=w529, "Y unit Out"="Hz" ("X unit"), "dB"=w526, "Y unit Curve"="%" ("Y unit"), "Y data  Curve"=u16 1 ("Y data"), "Lin"=w525, "dB ref Out"=w524, "dB ref Curve"=w523) -> (w530:T7)  [unwired: 2 in]
            n134 = Insert Into Array(array=w522, new element=T8 {"display X"=TRUE, "display Y"=TRUE, "display Z"=FALSE}) -> (w521:T3)  [unwired: 1 in]
            n135 = Insert Into Array(array=w532, new element=w530) -> (w531:T2[])  [unwired: 1 in]
          }
        }
      }
      frame 7 {
        n136 = Add(x=w544, y=10) -> (x+y=w542:i32)
        n137 = Index Array(array=w546, index=w542) -> (element=w549:string)
        n138 = case shown="True" w547 {
          tunnel: w548 -> [w552 w570]
          tunnel: w549 -> [_ w569]
          tunnel: [w552 w568] -> w545
          tunnel: w540 -> [w551 w567]
          tunnel: w539 -> [_ w564]
          tunnel: [w551 w566] -> w538
          tunnel: w537 -> [w550 w557]
          tunnel: [w550 w556] -> w536
          frame False {
          }
          frame True {
            n139 = Unbundle(w564) -> ("dB"=w561:u16, "Lin"=w560:u16, "dB ref Out"=w559:dbl, "dB ref Curve"=w558:dbl)  [unwired: 5 out]
            n140 = Insert Into Array(array=w570, new element=w569) -> (w568:string[])  [unwired: 1 in]
            n141 = Bundle(cluster=w564, "Y unit Out"="Hz" ("X unit"), "dB"=w561, "Y unit Curve"="%" ("Y unit"), "Y data  Curve"=u16 1 ("Y data"), "Y unit Curve"="deg." ("Z unit"), "Lin"=w560, "dB ref Out"=w559, "dB ref Curve"=w558) -> (w565:T7)  [unwired: 1 in]
            n142 = Insert Into Array(array=w557, new element=T8 {"display X"=TRUE, "display Y"=TRUE, "display Z"=FALSE}) -> (w556:T3)  [unwired: 1 in]
            n143 = Insert Into Array(array=w567, new element=w565) -> (w566:T2[])  [unwired: 1 in]
          }
        }
      }
      frame 8 {
        n144 = Add(x=w579, y=10) -> (x+y=w577:i32)
        n145 = Index Array(array=w581, index=w577) -> (element=w584:string)
        n146 = case shown="True" w582 {
          tunnel: w583 -> [w587 w605]
          tunnel: w584 -> [_ w604]
          tunnel: [w587 w603] -> w580
          tunnel: w575 -> [w586 w602]
          tunnel: w574 -> [_ w599]
          tunnel: [w586 w601] -> w573
          tunnel: w572 -> [w585 w592]
          tunnel: [w585 w591] -> w571
          frame False {
          }
          frame True {
            n147 = Unbundle(w599) -> ("dB"=w596:u16, "Lin"=w595:u16, "dB ref Out"=w594:dbl, "dB ref Curve"=w593:dbl)  [unwired: 5 out]
            n148 = Insert Into Array(array=w605, new element=w604) -> (w603:string[])  [unwired: 1 in]
            n149 = Bundle(cluster=w599, "Y unit Out"="Hz" ("X unit"), "dB"=w596, "Y unit Curve"="%" ("Y unit"), "Y data  Curve"=u16 1 ("Y data"), "Y unit Curve"="deg." ("Z unit"), "Lin"=w595, "dB ref Out"=w594, "dB ref Curve"=w593) -> (w600:T7)  [unwired: 1 in]
            n150 = Insert Into Array(array=w592, new element=T8 {"display X"=TRUE, "display Y"=TRUE, "display Z"=FALSE}) -> (w591:T3)  [unwired: 1 in]
            n151 = Insert Into Array(array=w602, new element=w600) -> (w601:T2[])  [unwired: 1 in]
          }
        }
      }
      frame 9 {
        n152 = Add(x=w614, y=10) -> (x+y=w612:i32)
        n153 = Index Array(array=w616, index=w612) -> (element=w619:string)
        n154 = case shown="True" w617 {
          tunnel: w618 -> [w622 w640]
          tunnel: w619 -> [_ w639]
          tunnel: [w622 w638] -> w615
          tunnel: w610 -> [w621 w637]
          tunnel: w609 -> [_ w634]
          tunnel: [w621 w636] -> w608
          tunnel: w607 -> [w620 w627]
          tunnel: [w620 w626] -> w606
          frame False {
          }
          frame True {
            n155 = Unbundle(w634) -> ("dB"=w631:u16, "Lin"=w630:u16, "dB ref Out"=w629:dbl, "dB ref Curve"=w628:dbl)  [unwired: 5 out]
            n156 = Insert Into Array(array=w640, new element=w639) -> (w638:string[])  [unwired: 1 in]
            n157 = Bundle(cluster=w634, "Y unit Out"="Hz" ("X unit"), "dB"=w631, "Y unit Curve"="%" ("Y unit"), "Y data  Curve"=u16 1 ("Y data"), "Y unit Curve"="deg." ("Z unit"), "Lin"=w630, "dB ref Out"=w629, "dB ref Curve"=w628) -> (w635:T7)  [unwired: 1 in]
            n158 = Insert Into Array(array=w627, new element=T8 {"display X"=TRUE, "display Y"=TRUE, "display Z"=FALSE}) -> (w626:T3)  [unwired: 1 in]
            n159 = Insert Into Array(array=w637, new element=w635) -> (w636:T2[])  [unwired: 1 in]
          }
        }
      }
      frame 10 {
        n160 = Add(x=w649, y=10) -> (x+y=w647:i32)
        n161 = Index Array(array=w651, index=w647) -> (element=w654:string)
        n162 = case shown="True" w652 {
          tunnel: w653 -> [w657 w675]
          tunnel: w654 -> [_ w674]
          tunnel: [w657 w673] -> w650
          tunnel: w645 -> [w656 w672]
          tunnel: w644 -> [_ w669]
          tunnel: [w656 w671] -> w643
          tunnel: w642 -> [w655 w662]
          tunnel: [w655 w661] -> w641
          frame False {
          }
          frame True {
            n163 = Unbundle(w669) -> ("dB"=w666:u16, "Lin"=w665:u16, "dB ref Out"=w664:dbl, "dB ref Curve"=w663:dbl)  [unwired: 5 out]
            n164 = Insert Into Array(array=w675, new element=w674) -> (w673:string[])  [unwired: 1 in]
            n165 = Bundle(cluster=w669, "Y unit Out"="Hz" ("X unit"), "dB"=w666, "Y unit Curve"="phons" ("Y unit"), "Y data  Curve"=u16 1 ("Y data"), "Y unit Curve"="deg." ("Z unit"), "Lin"=w665, "dB ref Out"=w664, "dB ref Curve"=w663) -> (w670:T7)  [unwired: 1 in]
            n166 = Insert Into Array(array=w662, new element=T8 {"display X"=TRUE, "display Y"=TRUE, "display Z"=FALSE}) -> (w661:T3)  [unwired: 1 in]
            n167 = Insert Into Array(array=w672, new element=w670) -> (w671:T2[])  [unwired: 1 in]
          }
        }
      }
      frame 11 {
        n168 = Add(x=w684, y=10) -> (x+y=w682:i32)
        n169 = Index Array(array=w686, index=w682) -> (element=w689:string)
        n170 = case shown="True" w687 {
          tunnel: w688 -> [w692 w709]
          tunnel: w689 -> [_ w708]
          tunnel: [w692 w707] -> w685
          tunnel: w680 -> [w691 w706]
          tunnel: w679 -> [_ w693]
          tunnel: [w691 w705] -> w678
          tunnel: w677 -> [w690 w698]
          tunnel: [w690 w697] -> w676
          frame False {
          }
          frame True {
            n171 = Unbundle(w693) -> ("dB"=w702:u16, "Lin"=w701:u16, "dB ref Out"=w700:dbl, "dB ref Curve"=w699:dbl)  [unwired: 5 out]
            n172 = Insert Into Array(array=w709, new element=w708) -> (w707:string[])  [unwired: 1 in]
            n173 = Bundle(cluster=w693, "Y unit Out"="Hz" ("X unit"), "dB"=w702, "Y unit Curve"="%" ("Y unit"), "Y data  Curve"=u16 1 ("Y data"), "Y unit Curve"="deg." ("Z unit"), "Lin"=w701, "dB ref Out"=w700, "dB ref Curve"=w699) -> ()  [unwired: 1 in, 1 out]
            n174 = Insert Into Array(array=w698, new element=T8 {"display X"=TRUE, "display Y"=TRUE, "display Z"=FALSE}) -> (w697:T3)  [unwired: 1 in]
            n175 = Insert Into Array(array=w706, new element=w693) -> (w705:T2[])  [unwired: 1 in]
          }
        }
      }
      frame 12 {
        n176 = Add(x=w718, y=10) -> (x+y=w716:i32)
        n177 = Index Array(array=w720, index=w716) -> (element=w723:string)
        n178 = case shown="True" w721 {
          tunnel: w722 -> [w726 w744]
          tunnel: w723 -> [_ w743]
          tunnel: [w726 w742] -> w719
          tunnel: w714 -> [w725 w741]
          tunnel: w713 -> [_ w738]
          tunnel: [w725 w740] -> w712
          tunnel: w711 -> [w724 w731]
          tunnel: [w724 w730] -> w710
          frame False {
          }
          frame True {
            n179 = Unbundle(w738) -> ("dB"=w735:u16, "Lin"=w734:u16, "dB ref Out"=w733:dbl, "dB ref Curve"=w732:dbl)  [unwired: 5 out]
            n180 = Insert Into Array(array=w744, new element=w743) -> (w742:string[])  [unwired: 1 in]
            n181 = Bundle(cluster=w738, "Y unit Out"="Hz" ("X unit"), "dB"=w735, "Y unit Curve"="%" ("Y unit"), "Y data  Curve"=u16 1 ("Y data"), "Y unit Curve"="deg." ("Z unit"), "Lin"=w734, "dB ref Out"=w733, "dB ref Curve"=w732) -> (w739:T7)  [unwired: 1 in]
            n182 = Insert Into Array(array=w731, new element=T8 {"display X"=TRUE, "display Y"=TRUE, "display Z"=FALSE}) -> (w730:T3)  [unwired: 1 in]
            n183 = Insert Into Array(array=w741, new element=w739) -> (w740:T2[])  [unwired: 1 in]
          }
        }
      }
      frame 13 {
        n184 = Add(x=w753, y=10) -> (x+y=w751:i32)
        n185 = Index Array(array=w755, index=w751) -> (element=w758:string)
        n186 = case shown="True" w756 {
          tunnel: w757 -> [w761 w779]
          tunnel: w758 -> [_ w778]
          tunnel: [w761 w777] -> w754
          tunnel: w749 -> [w760 w776]
          tunnel: w748 -> [_ w773]
          tunnel: [w760 w775] -> w747
          tunnel: w746 -> [w759 w766]
          tunnel: [w759 w765] -> w745
          frame False {
          }
          frame True {
            n187 = Unbundle(w773) -> ("dB"=w770:u16, "Lin"=w769:u16, "dB ref Out"=w768:dbl, "dB ref Curve"=w767:dbl)  [unwired: 5 out]
            n188 = Insert Into Array(array=w779, new element=w778) -> (w777:string[])  [unwired: 1 in]
            n189 = Bundle(cluster=w773, "Y unit Out"="Hz" ("X unit"), "dB"=w770, "Y unit Curve"="%" ("Y unit"), "Y data  Curve"=u16 1 ("Y data"), "Y unit Curve"="deg." ("Z unit"), "Lin"=w769, "dB ref Out"=w768, "dB ref Curve"=w767) -> (w774:T7)  [unwired: 1 in]
            n190 = Insert Into Array(array=w766, new element=T8 {"display X"=TRUE, "display Y"=TRUE, "display Z"=FALSE}) -> (w765:T3)  [unwired: 1 in]
            n191 = Insert Into Array(array=w776, new element=w774) -> (w775:T2[])  [unwired: 1 in]
          }
        }
      }
      frame 14 {
        n192 = Add(x=w788, y=10) -> (x+y=w786:i32)
        n193 = Index Array(array=w790, index=w786) -> (element=w793:string)
        n194 = case shown="True" w791 {
          tunnel: w792 -> [w796 w813]
          tunnel: w793 -> [_ w812]
          tunnel: [w796 w811] -> w789
          tunnel: w784 -> [w795 w810]
          tunnel: w783 -> [_ w797]
          tunnel: [w795 w809] -> w782
          tunnel: w781 -> [w794 w802]
          tunnel: [w794 w801] -> w780
          frame False {
          }
          frame True {
            n195 = Unbundle(w797) -> ("dB"=w806:u16, "Lin"=w805:u16, "dB ref Out"=w804:dbl, "dB ref Curve"=w803:dbl)  [unwired: 5 out]
            n196 = Insert Into Array(array=w813, new element=w812) -> (w811:string[])  [unwired: 1 in]
            n197 = Bundle(cluster=w797, "Y unit Out"="Hz" ("X unit"), "dB"=w806, "Y unit Curve"="%" ("Y unit"), "Y data  Curve"=u16 1 ("Y data"), "Y unit Curve"="deg." ("Z unit"), "Lin"=w805, "dB ref Out"=w804, "dB ref Curve"=w803) -> ()  [unwired: 1 in, 1 out]
            n198 = Insert Into Array(array=w802, new element=T8 {"display X"=TRUE, "display Y"=TRUE, "display Z"=FALSE}) -> (w801:T3)  [unwired: 1 in]
            n199 = Insert Into Array(array=w810, new element=w797) -> (w809:T2[])  [unwired: 1 in]
          }
        }
      }
      frame 15 {
        n200 = Add(x=w822, y=10) -> (x+y=w820:i32)
        n201 = Index Array(array=w824, index=w820) -> (element=w827:string)
        n202 = case shown="True" w825 {
          tunnel: w826 -> [w830 w848]
          tunnel: w827 -> [_ w847]
          tunnel: [w830 w846] -> w823
          tunnel: w818 -> [w829 w845]
          tunnel: w817 -> [_ w842]
          tunnel: [w829 w844] -> w816
          tunnel: w815 -> [w828 w835]
          tunnel: [w828 w834] -> w814
          frame False {
          }
          frame True {
            n203 = Unbundle(w842) -> ("dB"=w839:u16, "Lin"=w838:u16, "dB ref Out"=w837:dbl, "dB ref Curve"=w836:dbl)  [unwired: 5 out]
            n204 = Insert Into Array(array=w848, new element=w847) -> (w846:string[])  [unwired: 1 in]
            n205 = Bundle(cluster=w842, "Y unit Out"="Hz" ("X unit"), "dB"=w839, "Y unit Curve"="%" ("Y unit"), "Y data  Curve"=u16 1 ("Y data"), "Y unit Curve"="deg." ("Z unit"), "Lin"=w838, "dB ref Out"=w837, "dB ref Curve"=w836) -> (w843:T7)  [unwired: 1 in]
            n206 = Insert Into Array(array=w835, new element=T8 {"display X"=TRUE, "display Y"=TRUE, "display Z"=FALSE}) -> (w834:T3)  [unwired: 1 in]
            n207 = Insert Into Array(array=w845, new element=w843) -> (w844:T2[])  [unwired: 1 in]
          }
        }
      }
      frame 16 {
        n208 = Add(x=w857, y=10) -> (x+y=w855:i32)
        n209 = Index Array(array=w859, index=w855) -> (element=w862:string)
        n210 = case shown="True" w860 {
          tunnel: w861 -> [w865 w883]
          tunnel: w862 -> [_ w882]
          tunnel: [w865 w881] -> w858
          tunnel: w853 -> [w864 w880]
          tunnel: w852 -> [_ w877]
          tunnel: [w864 w879] -> w851
          tunnel: w850 -> [w863 w870]
          tunnel: [w863 w869] -> w849
          frame False {
          }
          frame True {
            n211 = Unbundle(w877) -> ("dB"=w874:u16, "Lin"=w873:u16, "dB ref Out"=w872:dbl, "dB ref Curve"=w871:dbl)  [unwired: 5 out]
            n212 = Insert Into Array(array=w883, new element=w882) -> (w881:string[])  [unwired: 1 in]
            n213 = Bundle(cluster=w877, "Y unit Out"="Hz" ("X unit"), "dB"=w874, "Y unit Curve"="%" ("Y unit"), "Y data  Curve"=u16 1 ("Y data"), "Y unit Curve"="deg." ("Z unit"), "Lin"=w873, "dB ref Out"=w872, "dB ref Curve"=w871) -> (w878:T7)  [unwired: 1 in]
            n214 = Insert Into Array(array=w870, new element=T8 {"display X"=TRUE, "display Y"=TRUE, "display Z"=FALSE}) -> (w869:T3)  [unwired: 1 in]
            n215 = Insert Into Array(array=w880, new element=w878) -> (w879:T2[])  [unwired: 1 in]
          }
        }
      }
    }
  }
  "Harmonics Orders Out" <- w41
  "Display Array" <- w27
  "Unit Info Out" <- w30
  n216 = call "CRYGet Real CurveName.vi"("Key No"=2, "Additive Info"="Additive Info", "CurveArrayByType"=w14) -> ("Curve Info Array Out"=→"Curve Info Array Out":T1)  [unwired: 8 in]
